vi "TDC.vi"(0 "sync.resources":T1, 1 "sync.Reference Clock":bool, 2 "sync.meas.oversample clock":refnum<k21>, 7 "sync.meas.arm":bool, 9 "sync.cptr":bool) -> (4 "sync.resources":T1, 6 "count out":u16, 8 "count valid":bool, 10 "rollover error":bool, 15 "measurement done (rising edge)":bool)   [LabVIEW 2013, in "ni579x Synchronization v1 FPGA.lvlib"]
doc: "This TDC VI will count the amount of time between two input signals. The 'time' is in units of 1/2 fast clocks, which is referred to as the oversample rate. The oversample clock is 1.5x the sample clock. Therefore, if the oversample clock is 300 MHz, the count will be the number of 600 MHz clocks seen. The oversample rate will be 3x (600 MHz vs 200 MHz).\n\nThe VI measures the time between the reference and the 'signal to measure'. Once the VI is enabled and has been armed, it will begin counting when it sees a rising edge of the reference. It will finish counting when it sees a rising edge of the 'signal to measure'."
uses:
  <instrlib>/ni579x/Synchronization/v1/FPGA/ni579x Synchronization v1 FPGA.lvlib
  <instrlib>/ni579x/Synchronization/v1/FPGA/Implementation/Resources.ctl
  <vilib>/rvi/IPIntegrationNode/IPINode_Utilities/niFpgaIPINodeSimCore.vi
  <vilib>/rvi/IPIntegrationNode/IPINode_Xnode/niFpgaIPINode.xnode
  <instrlib>/ni579x/Synchronization/v1/FPGA/Implementation/TDCSimFiles/Tdc_B556FC327CC64155836DD41C31E521AC.dll
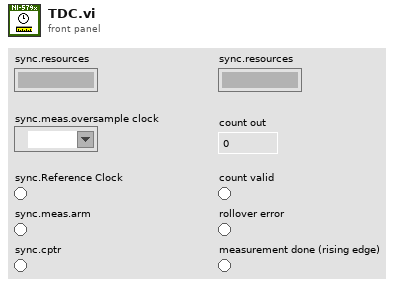
[diagram p1: front panel]
types:
  T1 = typedef "ni579x Synchronization v1 FPGA.lvlib/Resources.ctl" = cluster{"master":refnum<k21>, "meas.enable":refnum<k21>, "meas.ready":refnum<k21>, "meas.arm":refnum<k21>, "meas.valid":refnum<k21>, "meas.value":refnum<k21>, "meas.oversample clock":refnum<k21>, "meas.oversample factor":refnum<k21>, "cptr":refnum<k21>, "cptr.adjust":refnum<k21>, "cptr.period":refnum<k21>}
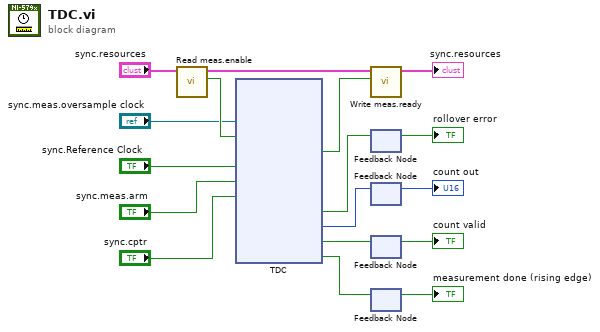
[diagram p0: block diagram]
diagram:
  n1 = call <instrlib>:"Read meas.enable.vi"("sync.resources"="sync.resources") -> ("meas.enable"=w6:bool, "sync.resources"=w4:T1)  [unwired: 9 in]
  n2 = xnode ("TDC")("derived clock"="sync.meas.oversample clock", "senablemeas"=w6, "atimerefin"="sync.Reference Clock", "aarmcounter"="sync.meas.arm", "strigenin"="sync.cptr") -> ("sreadytomeas"=w5:bool, "srollovererr"=w10:bool, "scountout"=w9:u16, "scountvalid"=w8:bool, "smeasdonere"=w7:bool)
  n3 = call <instrlib>:"Write meas.ready.vi"("meas.ready"=w5, "sync.resources"=w4) -> ("sync.resources"=→"sync.resources":T1)  [unwired: 9 in]
  n4 = feedback #1() -> (→"rollover error":bool)  [unwired: 1 in]
  n5 = feedback-in #1(w10) -> ()
  n6 = feedback #2() -> (→"count out":u16)  [unwired: 1 in]
  n7 = feedback-in #2(w9) -> ()
  n8 = feedback #3() -> (→"count valid":bool)  [unwired: 1 in]
  n9 = feedback-in #3(w8) -> ()
  n10 = feedback #4() -> (→"measurement done (rising edge)":bool)  [unwired: 1 in]
  n11 = feedback-in #4(w7) -> ()
